vi "from CDATA.vi"(3 "CDATA String":string) -> (11 "String in":string)   [LabVIEW 2010]
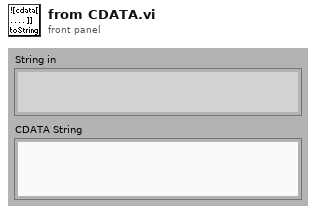
[diagram p1: front panel]
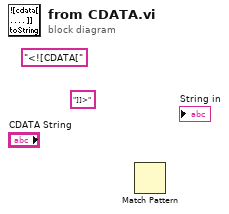
[diagram p0: block diagram]
diagram:
  (unwired) "]]>" ("format string")
  (unwired) "<![CDATA[" ("format string")
  n1 = Match Pattern() -> ()  [unwired: 3 in, 4 out]
